vi "Joystick and Camera move - external Connection.vi"(0 "Motion in":refnum<class "Motion.lvclass">, 1 "XYZTheta":dbl[](array[numeric]), 2 "Measurement Point":string, 3 "Inital GO":bool=TRUE) -> (7 "Motion out":refnum<class "Motion.lvclass">, 8 "Sum":dbl[](array[numeric]), 9 "Gantry":dbl[](array[numeric]), 10 "error out":errorcluster)   [LabVIEW 2016]
uses:
  Classes/Controllers/Camera/Copy of Camera Folder/Machine Vision.ctl
  Classes/Controllers/Motion/Copy of Motion Folder/Motion.lvclass
  Classes/Controllers/Camera/Copy of Camera Folder/Camera.lvclass
panel:
  out "fitting radius":dbl[](array[numeric])
  in  "Machine Vision 2":T1=enum."None"
  out "Image 2":T2(plugin-control)
  out "Focus Index":dbl[](array[numeric])
  in  "interval":dbl=0.005
  out "Score":dbl[](array[numeric])
  out "Waveform Graph":dbl[](graph)
  in  "focus":bool
  out "Numeric":dbl
  in  "Go SUM":bool
  in  "Z Go":bool
  in  "Position":dbl
  in  "Machine Vision":T1
  in  "Go":bool
  in  "Joystick":bool
  in  "Stop":bool
  out "Image":T2(plugin-control)
  out "Camera":dbl[](array[numeric])
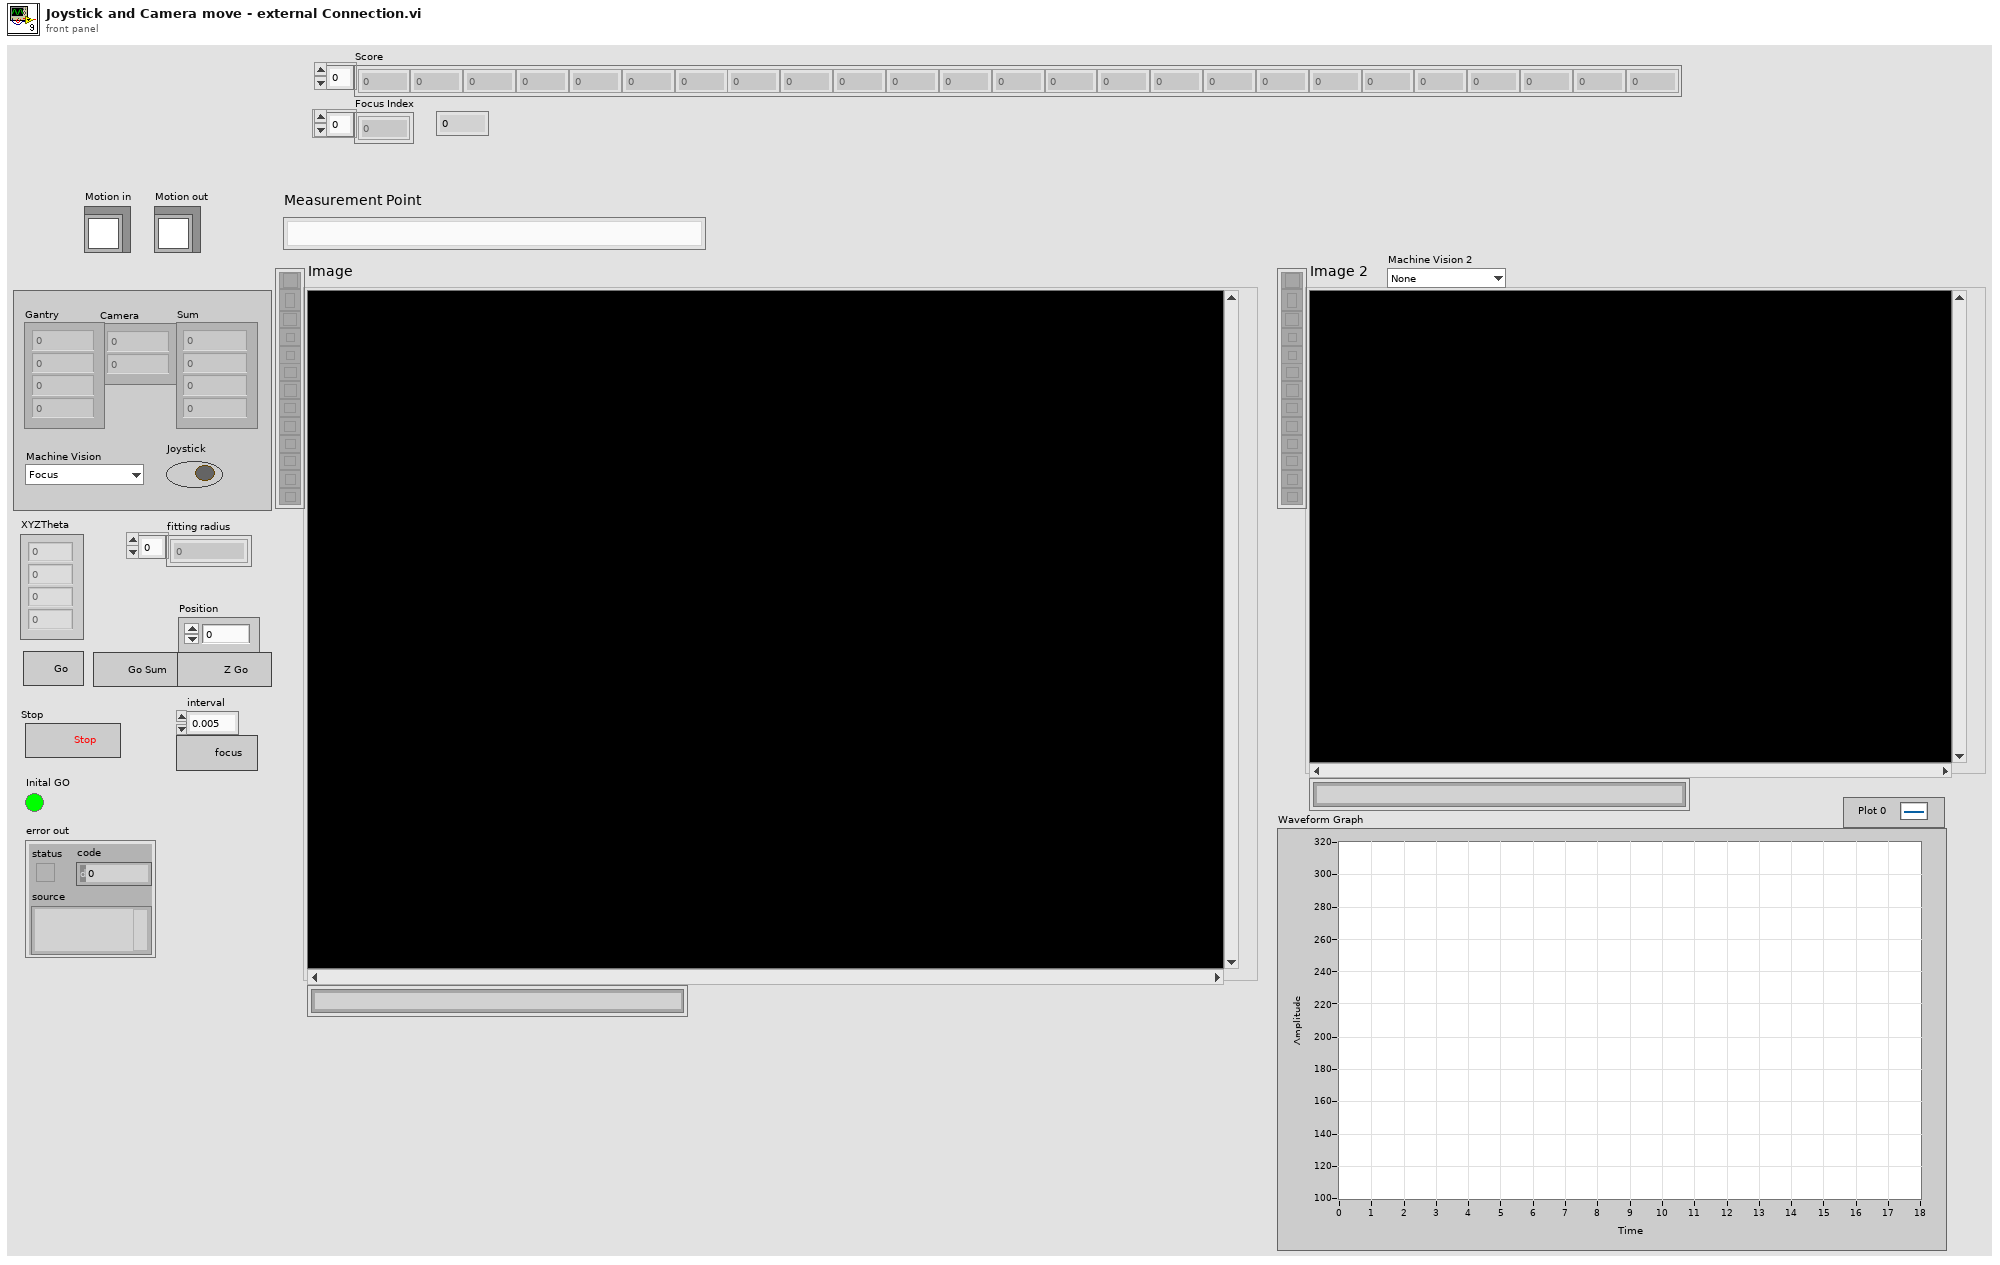
[diagram p1: front panel]
types:
  T1 = typedef "Camera.lvclass/Machine Vision.ctl" = enum16{"Focus", "LargeCircle", "None", "INTT HDI Mark", "INTT Sensor Cross", "INTT Chip Corner", "HPK Silicon", "circle"}
  T2 = typedef "IMAQ Image.ctl" = refnum<image>
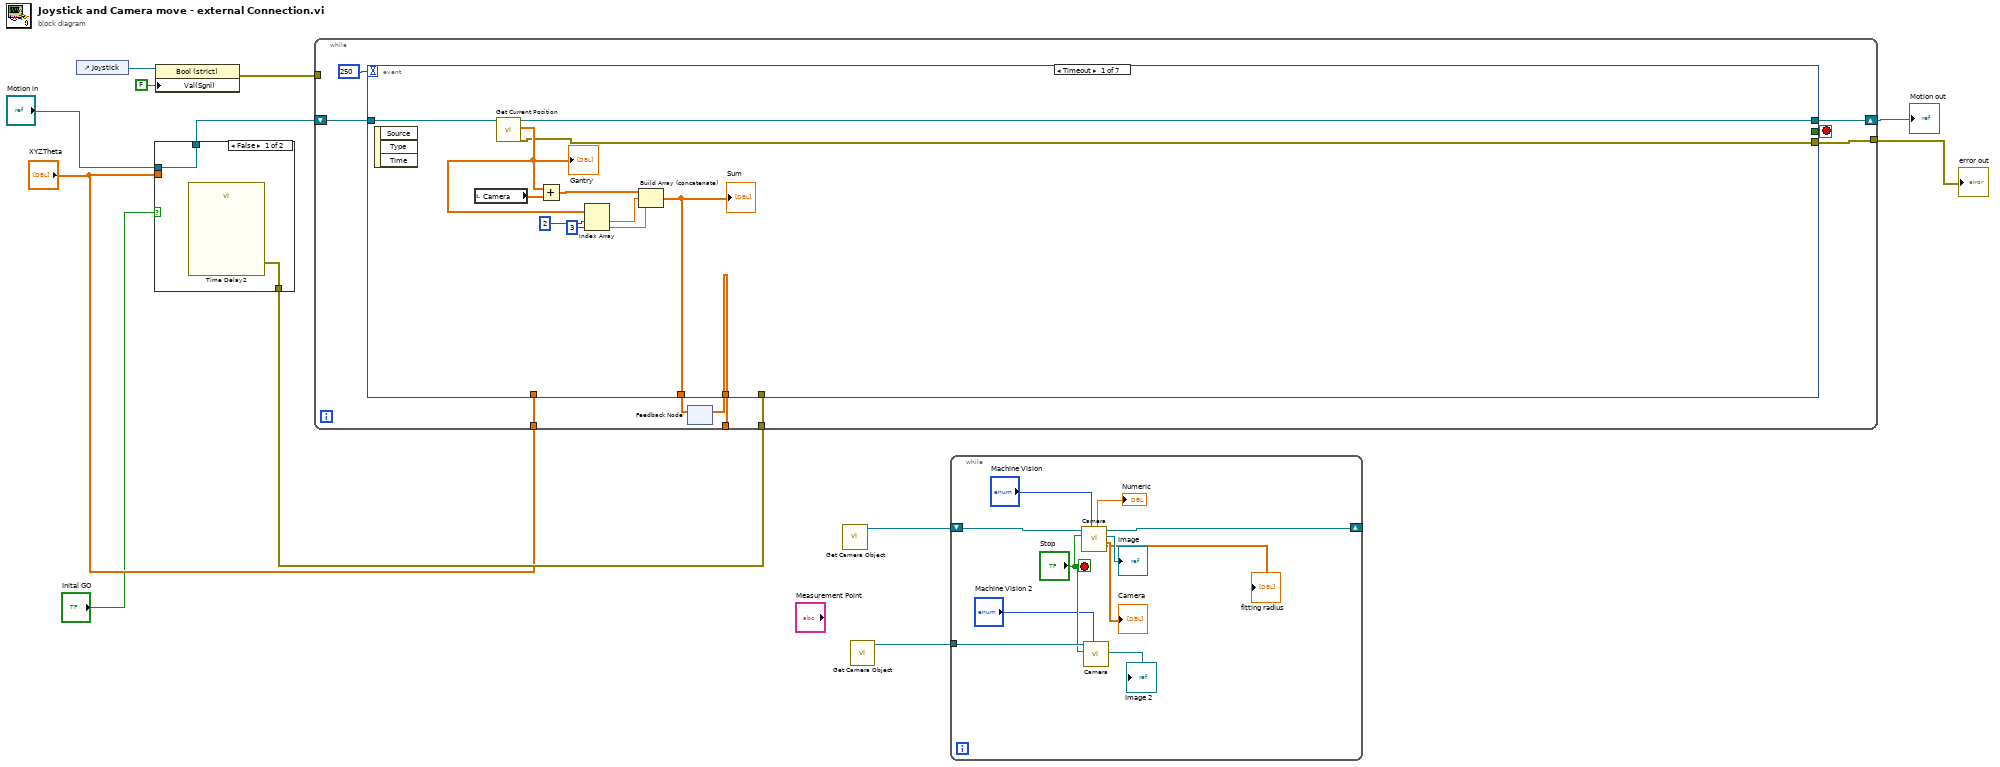
[diagram p0: block diagram]
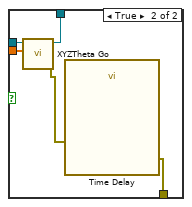
[diagram p2: hidden frame]
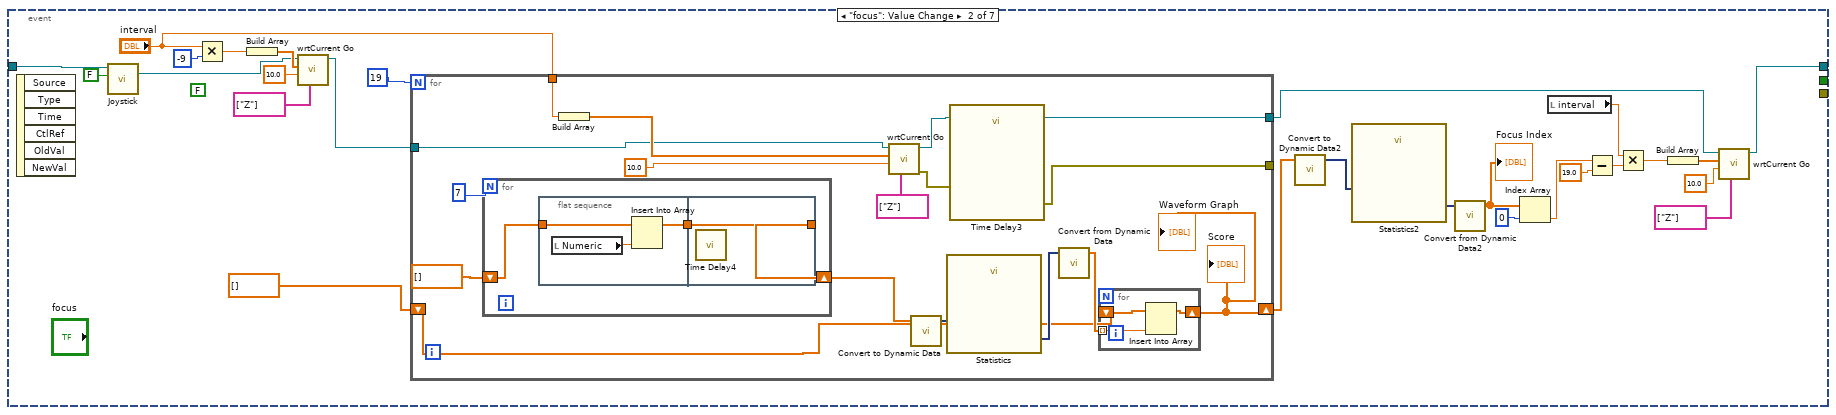
[diagram p3: hidden frame]
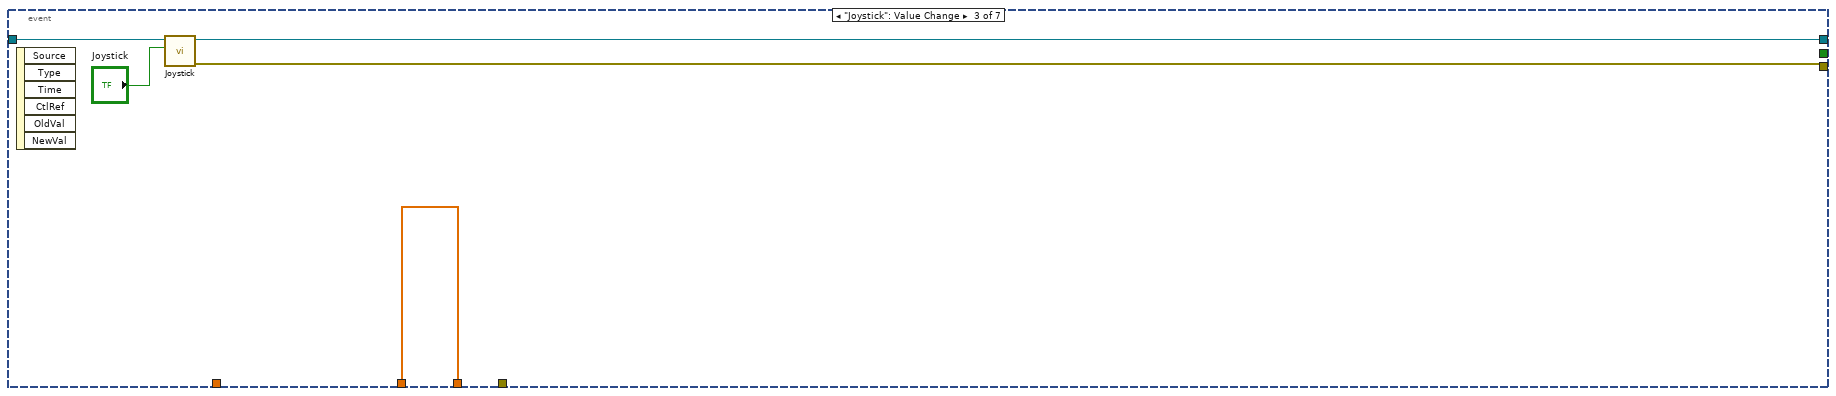
[diagram p4: hidden frame]
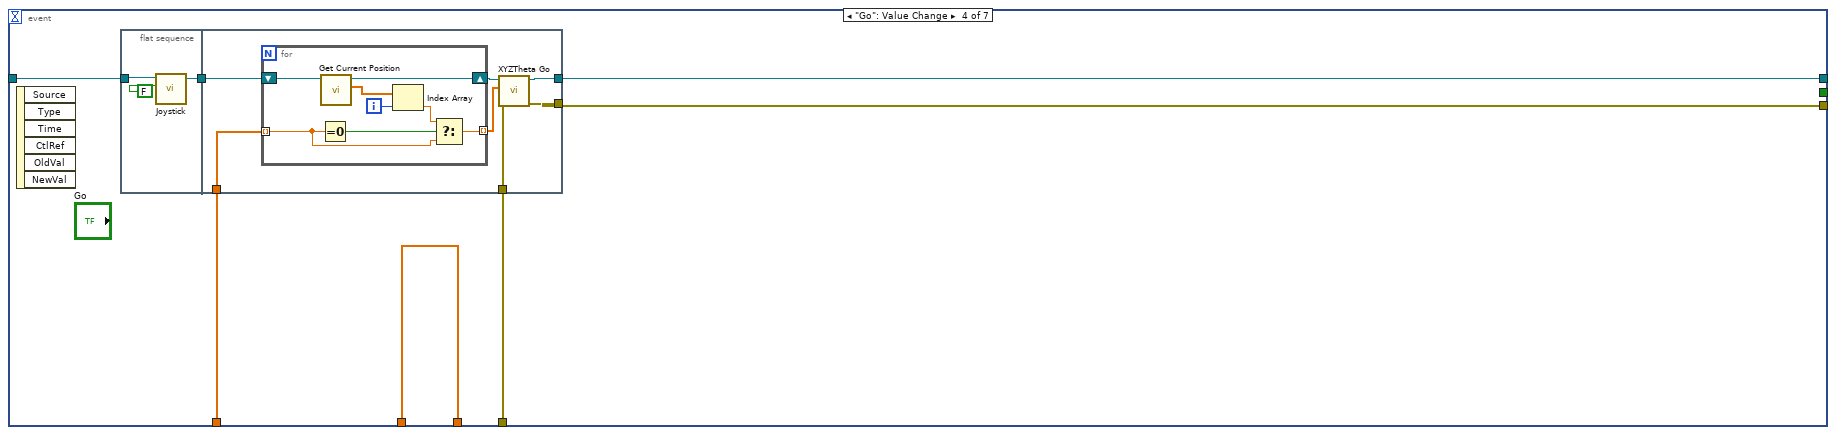
[diagram p5: hidden frame]
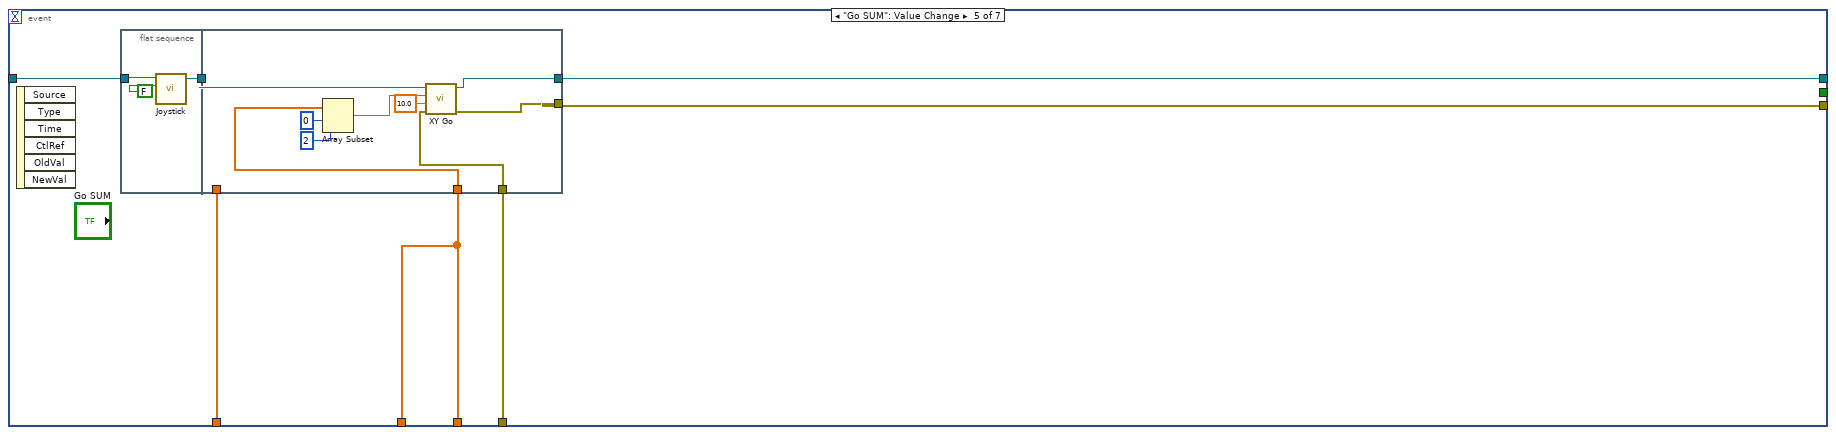
[diagram p6: hidden frame]
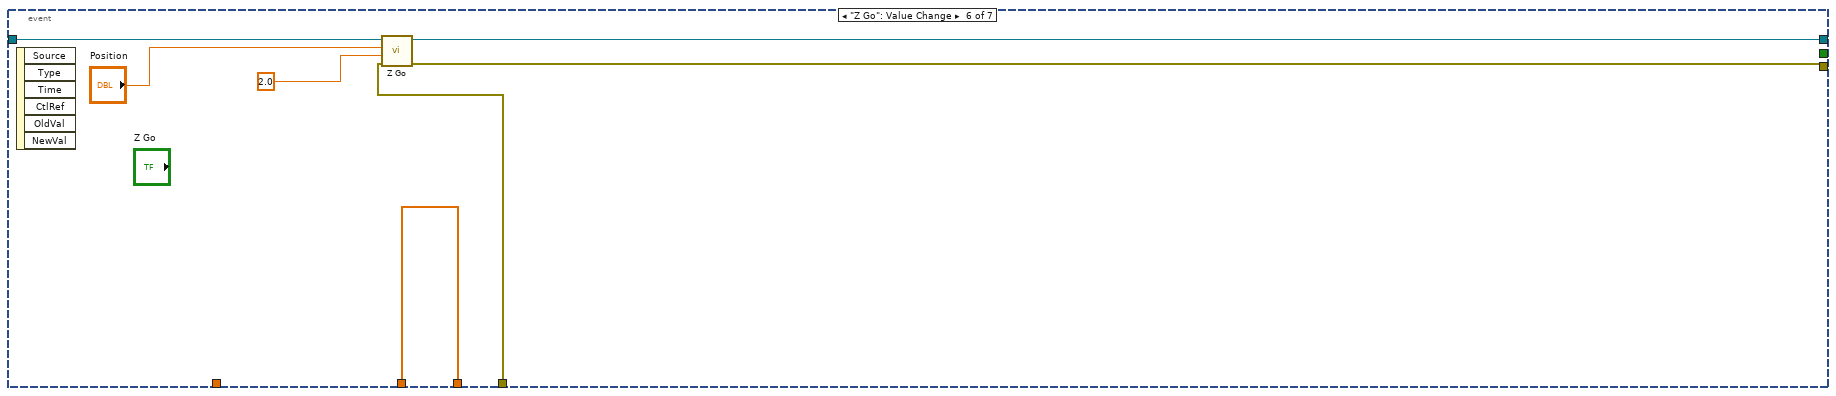
[diagram p7: hidden frame]
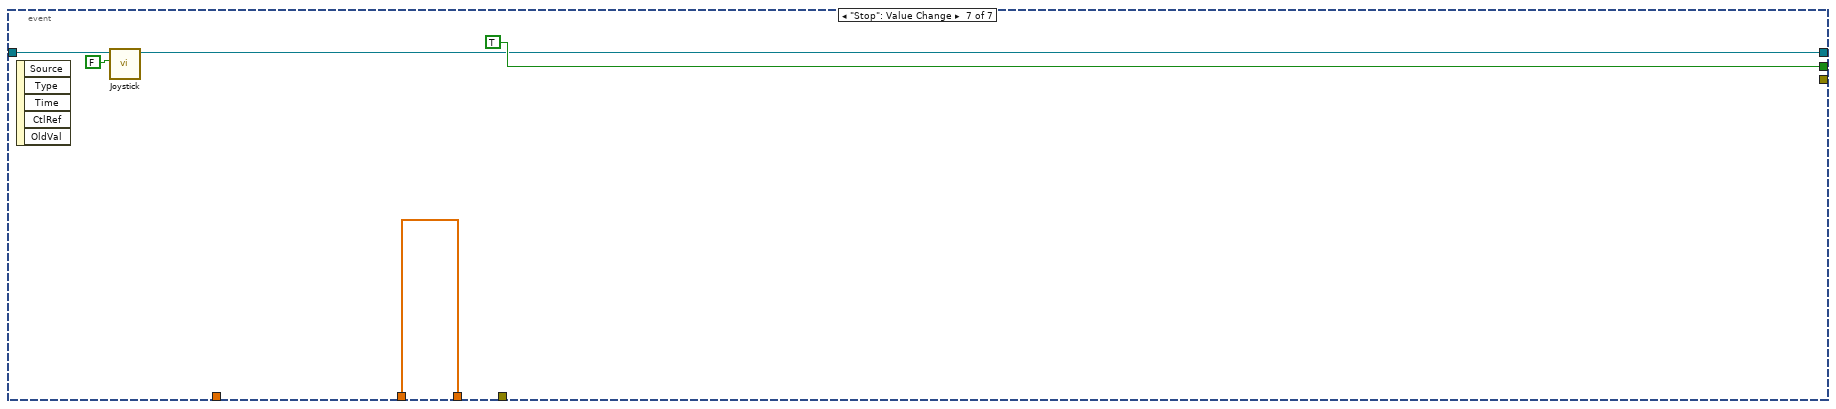
[diagram p8: hidden frame]
diagram:
  n1 = control-ref of="Joystick"() -> (w11:refnum<vi>)
  n2 = case shown="False" "Inital GO" {
    tunnel: "Motion in" -> [w14 w19]
    tunnel: [w14 w18] -> w5
    tunnel: [w13 w16] -> w4
    tunnel: "XYZTheta" -> [_ w15]
    frame False {
      n3 = call "Time Delay2"() -> ("error out"=w13:errorcluster)  [unwired: 11 in]
    }
    frame True {
      n4 = call "XYZTheta Go.vi"("XYZTheta In"=w15, "Motion in"=w19) -> ("error out"=w17:errorcluster, "Motion out"=w18:refnum<class "Motion.lvclass">)  [unwired: 7 in, 1 out]
      n5 = call "Time Delay"("error in (no error)"=w17) -> ("error out"=w16:errorcluster)  [unwired: 10 in]
    }
  }
  n6 = property class="Bool (strict)"(reference=w11, "Val(Sgnl)"=FALSE ("Value (Signaling)")) -> (error out=w10:errorcluster)  [unwired: 1 in, 1 out]
  n7 = while {
    shift-right: [w25] -> w8
    shift-left: w5 -> [w26]
    tunnel: w10 -> [_]
    tunnel: [w24] -> w7
    tunnel: w4 -> [w23]
    tunnel: "XYZTheta" -> [w22]
    tunnel: [w20] -> _
    stop <- w27 stop-if-true
    n8 = feedback #1() -> (w20:dbl[])  [unwired: 1 in]
    n9 = event shown="[0] Timeout" {
      selector: _ -> [_ _ _ _ _ _ _]
      dyn-events: _ -> [_ _ _ _ _ _ _]
      timeout: 250 -> [_ _ _ _ _ _ _]
      tunnel: [_ _ _ _ _ _ TRUE] -> w27
      tunnel: w26 -> [w38 w42 w97 w104 w129 w148 w152]
      tunnel: [w37 w41 w95 w103 w124 w147 w150] -> w25
      tunnel: [w32 _ w94 w101 w127 w142 _] -> w24
      tunnel: w23 -> [_ _ _ w100 w126 w143 _]
      tunnel: w22 -> [_ _ _ w99 w125 _ _]
      tunnel: [w29 _ w93 w98 w123 w144 w149] -> w21
      tunnel: w20 -> [_ _ w93 w98 w123 w144 w149]
      event Timeout {
        n10 = event-data() -> ()  [unwired: 1 in, 3 out]
        n11 = local read "Camera"() -> (w39:dbl[])
        n12 = call-dynamic "Get Current Position.vi"("Motion in"=w38) -> ("error out"=w32:errorcluster, "XYZTheta Out"=w35:dbl[], "Motion out"=w37:refnum<class "Motion.lvclass">)  [unwired: 8 in]
        "Gantry" <- w35
        n13 = Add(x=w35, y=w39) -> (x+y=w36:dbl[])
        n14 = Index Array(array=w35, index #1=2 ("index"), index #2=3 ("index")) -> (element #1=w33:dbl, element #2=w30:dbl)
        n15 = Build Array (concatenate)(w36, w33, w30) -> (w29:dbl[])
        "Sum" <- w29
      }
      event "focus": Value Change {
        (unwired) FALSE ("Joystick")
        n16 = event-data() -> ()  [unwired: 1 in, 6 out]
        n17 = call-dynamic "Joystick.vi"("Joystick"=FALSE, "Motion in"=w42) -> ("Motion out"=w44:refnum<class "Motion.lvclass">)  [unwired: 8 in, 1 out]
        n18 = Multiply(x="interval", y=-9) -> (x*y=w59:dbl)
        n19 = Build Array(w59) -> (w61:dbl[])
        n20 = call-dynamic "wrtCurrent Go.vi"("axis names"=string[] ["Z"] ("Axis"), "Speed"=10.0, "distances"=w61, "Motion in"=w44) -> ("Motion out"=w65:refnum<class "Motion.lvclass">)  [unwired: 6 in, 1 out]
        n21 = for {
          N: 19 -> [_]
          tunnel: w65 -> [w67]
          tunnel: [w71] -> w51
          shift-right: [w68] -> w57
          shift-left: dbl[] [] -> [w69]
          tunnel: "interval" -> [w74]
          tunnel: [w70] -> _
          n22 = for {
            N: 7 -> [_]
            shift-right: [w88] -> w79
            shift-left: dbl[] [] -> [w87]
            n23 = flat-sequence {
              tunnel: w87 -> [w90]
              tunnel: [w91] -> w86
              tunnel: [w92] -> w88
              tunnel: w86 -> [w92]
              frame #0 {
                n24 = local read "Numeric"() -> (w89:dbl)
                n25 = Insert Into Array(array=w90, new element=w89) -> (w91:dbl[])  [unwired: 1 in]
              }
              frame #1 {
                n26 = call "Time Delay4"() -> ()  [unwired: 11 in, 1 out]
              }
            }
          }
          n27 = Build Array(w74) -> (w73:dbl[])
          n28 = call-dynamic "wrtCurrent Go.vi"("axis names"=string[] ["Z"] ("Axis"), "Speed"=10.0, "distances"=w73, "Motion in"=w67) -> ("error out"=w80:errorcluster, "Motion out"=w71:refnum<class "Motion.lvclass">)  [unwired: 6 in]
          n29 = call "Convert to Dynamic Data"("Array"=w79) -> ("Dynamic Data Type"=w78:dynamicdata)  [unwired: 3 in]
          n30 = call "Statistics"("Signals"=w78) -> ("Arithmetic Mean"=w76:dynamicdata)  [unwired: 25 in, 1 out]
          n31 = call "Time Delay3"("error in (no error)"=w80) -> ("error out"=w70:errorcluster)  [unwired: 10 in]
          n32 = call "Convert from Dynamic Data"("Dynamic Data Type"=w76) -> ("Array"=w72:dbl[])  [unwired: 3 in]
          n33 = for {
            tunnel: w72 -> [w85] mode=indexing
            shift-right: [w84] -> w68
            shift-left: w69 -> [w83]
            n34 = Insert Into Array(array=w83, new element=w85) -> (w84:dbl[])  [unwired: 1 in]
          }
          "Score" <- w68
          "Waveform Graph" <- w68
        }
        n35 = call "Convert to Dynamic Data2"("Array"=w57) -> ("Dynamic Data Type"=w56:dynamicdata)  [unwired: 3 in]
        n36 = call "Statistics2"("Signals"=w56) -> ("Index of Max"=w55:dynamicdata)  [unwired: 25 in, 1 out]
        n37 = call "Convert from Dynamic Data2"("Dynamic Data Type"=w55) -> ("Array"=w43:dbl[])  [unwired: 3 in]
        "Focus Index" <- w43
        n38 = Index Array(array=w43, index=0) -> (element=w46:dbl)
        n39 = local read "interval"() -> (w49:dbl)
        n40 = Subtract(x=w46, y=19.0 ("x")) -> (x-y=w50:dbl)
        n41 = Multiply(x=w49, y=w50) -> (x*y=w48:dbl)
        n42 = Build Array(w48) -> (w47:dbl[])
        n43 = call-dynamic "wrtCurrent Go.vi"("axis names"=string[] ["Z"] ("Axis"), "Speed"=10.0, "distances"=w47, "Motion in"=w51) -> ("Motion out"=w41:refnum<class "Motion.lvclass">)  [unwired: 6 in, 1 out]
      }
      event "Joystick": Value Change {
        n44 = event-data() -> ()  [unwired: 1 in, 6 out]
        n45 = call-dynamic "Joystick.vi"("Joystick"="Joystick", "Motion in"=w97) -> ("error out"=w94:errorcluster, "Motion out"=w95:refnum<class "Motion.lvclass">)  [unwired: 8 in]
      }
      event "Go": Value Change {
        n46 = event-data() -> ()  [unwired: 1 in, 6 out]
        n47 = flat-sequence {
          tunnel: w104 -> [w106]
          tunnel: [w105] -> w102
          tunnel: [w111] -> w103
          tunnel: w102 -> [w114]
          tunnel: [w110] -> w101
          tunnel: w100 -> [w109]
          tunnel: w99 -> [w108]
          frame #0 {
            n48 = call-dynamic "Joystick.vi"("Joystick"=FALSE, "Motion in"=w106) -> ("Motion out"=w105:refnum<class "Motion.lvclass">)  [unwired: 8 in, 1 out]
          }
          frame #1 {
            n49 = for {
              tunnel: w108 -> [w120] mode=indexing
              tunnel: [w118] -> w113 mode=indexing
              shift-right: [w116] -> w112
              shift-left: w114 -> [w117]
              i -> [w122]
              n50 = Equal To 0?(x=w120) -> (x = 0?=w121:bool)
              n51 = call-dynamic "Get Current Position.vi"("Motion in"=w117) -> ("XYZTheta Out"=w115:dbl[], "Motion out"=w116:refnum<class "Motion.lvclass">)  [unwired: 8 in, 1 out]
              n52 = Index Array(array=w115, index=w122) -> (element=w119:dbl)
              n53 = Select(t=w119, s=w121, f=w120) -> (s? t:f=w118:dbl)
            }
            n54 = call "XYZTheta Go.vi"("error in (no error)"=w109, "XYZTheta In"=w113, "Motion in"=w112) -> ("error out"=w110:errorcluster, "Motion out"=w111:refnum<class "Motion.lvclass">)  [unwired: 6 in, 1 out]
          }
        }
      }
      event "Go SUM": Value Change {
        n55 = event-data() -> ()  [unwired: 1 in, 6 out]
        n56 = flat-sequence {
          tunnel: w129 -> [w131]
          tunnel: [w130] -> w128
          tunnel: w128 -> [w137]
          tunnel: [w135] -> w127
          tunnel: w126 -> [w136]
          tunnel: w125 -> [_]
          tunnel: w123 -> [w140]
          tunnel: [w134] -> w124
          frame #0 {
            n57 = call-dynamic "Joystick.vi"("Joystick"=FALSE, "Motion in"=w131) -> ("Motion out"=w130:refnum<class "Motion.lvclass">)  [unwired: 8 in, 1 out]
          }
          frame #1 {
            n58 = Array Subset(array=w140, index=0, length=2) -> (w133:dbl[])
            n59 = call-dynamic "XY Go.vi"("error in (no error)"=w136, "Speed"=10.0, "XY"=w133, "Motion in"=w137) -> ("error out"=w135:errorcluster, "Motion out"=w134:refnum<class "Motion.lvclass">)  [unwired: 6 in]
          }
        }
      }
      event "Z Go": Value Change {
        n60 = event-data() -> ()  [unwired: 1 in, 6 out]
        n61 = call-dynamic "Z Go.vi"("error in (no error)"=w143, "Speed"=2.0, "Position"="Position", "Motion in"=w148) -> ("error out"=w142:errorcluster, "Motion out"=w147:refnum<class "Motion.lvclass">)  [unwired: 6 in]
      }
      event "Stop": Value Change {
        n62 = event-data() -> ()  [unwired: 1 in, 5 out]
        n63 = call-dynamic "Joystick.vi"("Joystick"=FALSE, "Motion in"=w152) -> ("Motion out"=w150:refnum<class "Motion.lvclass">)  [unwired: 8 in, 1 out]
      }
    }
    n64 = feedback-in #1(w21) -> ()
  }
  "error out" <- w7
  "Motion out" <- w8
  n65 = call "Get Camera Object.vi"() -> ("Camera out"=w9:refnum<class "Camera.lvclass">)  [unwired: 10 in, 1 out]
  n66 = call "Get Camera Object.vi"() -> ("Camera out"=w1:refnum<class "Camera.lvclass">)  [unwired: 10 in, 1 out]
  n67 = while {
    shift-right: [w163] -> _
    shift-left: w9 -> [w164]
    tunnel: w1 -> [w158]
    stop <- "Stop" stop-if-true
    n68 = call "Camera.vi"("Machine Vision"="Machine Vision", "Stop"="Stop", "Camera in"=w164) -> ("Camera"=→"Camera":dbl[], "Image"=→"Image":T2, "Camera out"=w163:refnum<class "Camera.lvclass">, "Numeric"=→"Numeric":dbl, "camera R"=→"fitting radius":dbl[])  [unwired: 2 in, 2 out]
    n69 = call "Camera.vi"("Machine Vision"="Machine Vision 2", "Stop"="Stop", "Camera in"=w158) -> ("Image"=→"Image 2":T2)  [unwired: 2 in, 6 out]
  }
